vi "Zero-Order Hold.vi"   [LabVIEW 2017, in "NI_AdvCtrl_discrete linear.lvlib"]
doc: "LabVIEW no longer supports this VI. You can obtain similar functionality by installing the LabVIEW Simulation Module.\n\nHolds the signal for a definite period of time. In other words, the prediction of the signal is based only on the current input point."
uses:
  <vilib>/addons/control/advanced/NI_AdvCtrl_discrete linear.lvlib
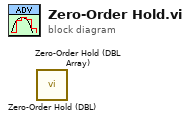
[diagram p0: block diagram]
diagram:
  n1 = call <vilib>:"Zero-Order Hold (DBL).vi"() -> ()  [unwired: 5 in, 1 out]
  n2 = call <vilib>:"Zero-Order Hold (DBL Array).vi"() -> ()  [unwired: 5 in, 1 out]
